vi "FTW-Socket-Core-LibraryError.vi"(0 "error in":errorcluster, 7 "Return Value":i64) -> (4 "error out":errorcluster)   [LabVIEW 2014]
uses:
  error/FTW-ERR-ThrowGenericError.vi
  error/FTW-ERR-NoErrorConstant.vi
  error/FTW-ERR-CallChain.vi
  string/FTW-STR-ReplaceWhitespace.vi
panel:
  # "Inputs"
  # "Outputs"
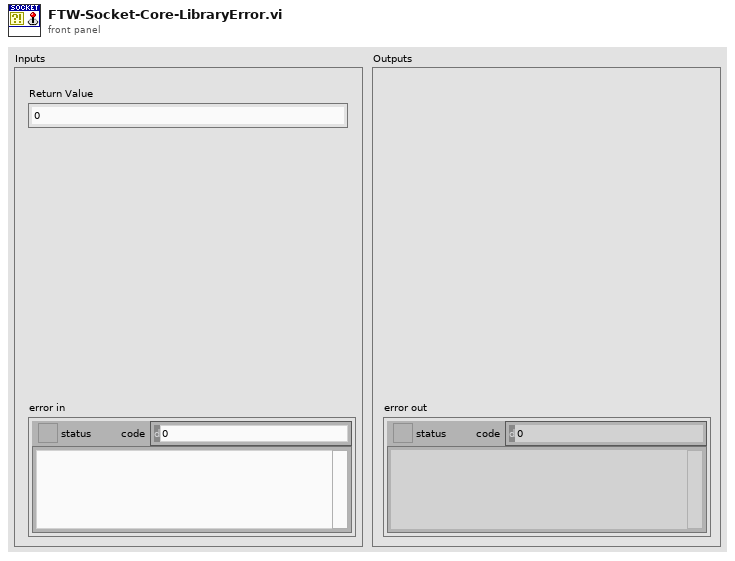
[diagram p1: front panel]
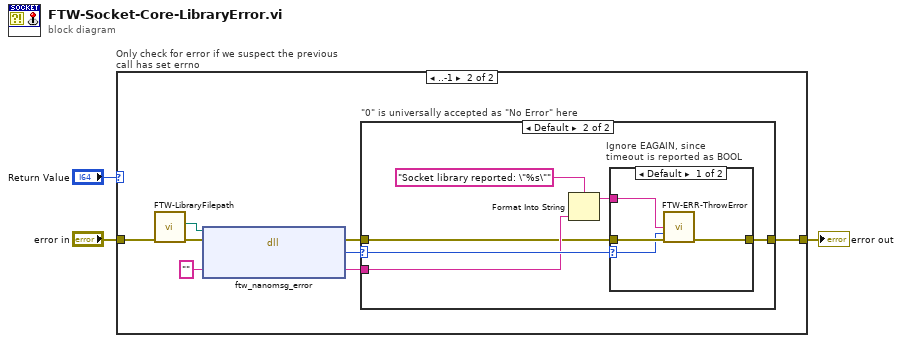
[diagram p0: block diagram]
diagram:
  n1 = case "Only check for error if we suspect the previous call has set errno" shown="..-1" "Return Value" {
    tunnel: [w4 w12] -> w3
    tunnel: "error in" -> [w4 w9]
    frame 0.. {
    }
    frame ..-1 {
      n2 = call "FTW-LibraryFilepath.vi"("error in"=w9) -> ("error out"=w8:errorcluster, "Library Filepath"=w7:path)  [unwired: 8 in, 1 out]
      n3 = dll-call lib="?" fn="ftw_nanomsg_error"(path in=w7, error in=w8, "Message"="") -> (error out=w11:errorcluster, "Error Code"=w10:i32, "Message"=w5:string)  [unwired: 1 in, 1 out]
      n4 = case "\"0\" is universally accepted as \"No Error\" here" shown="Default" w10 {
        selector: w10 -> [_ w16]
        tunnel: w11 -> [w13 w14]
        tunnel: [w13 w19] -> w12
        tunnel: w5 -> [_ w15]
        frame 0 {
        }
        frame Default {
          n5 = Format Into String(format string="Socket library reported: \"%s\"" ("Error Message"), w15) -> (resulting string=w17:string)  [unwired: 2 in, 1 out]
          n6 = case "Ignore EAGAIN, since\ntimeout is reported as BOOL" shown="Default" w16 {
            selector: w16 -> [w20 _]
            tunnel: w14 -> [w23 w24]
            tunnel: [w22 w24] -> w19
            tunnel: w17 -> [w21 _]
            frame Default {
              n7 = call "FTW-ERR-ThrowError.vi"("Error Message"=w21, "Error Code"=w20, "error in"=w23) -> ("error out"=w22:errorcluster)  [unwired: 12 in]
            }
            frame 11 {
            }
          }
        }
      }
    }
  }
  "error out" <- w3
